vi "PID DAQ Multi-Channel UI Update.vi"(7 "Sample Data":dbl[][](array[numeric]), 8 "error in":errorcluster, 10 "Sample Parameter":variant[](array[variant]), 11 "Sample Number":i32) -> (0 "error out":errorcluster)   [LabVIEW 2011]
uses:
  Controls/User Interface Action.ctl
  Functional Global Data/Run Data.ctl
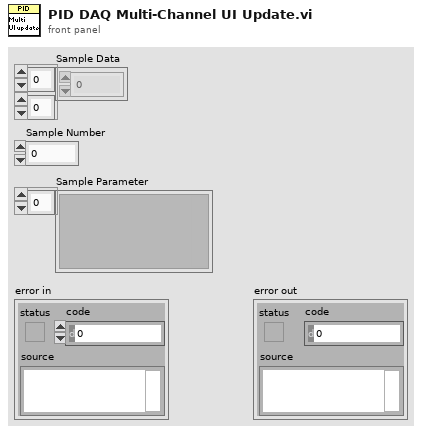
[diagram p1: front panel]
types:
  T1 = typedef "User Interface Action.ctl" = enum16{"Initialize", "Data Acquisition Disable", "Data View Disable", "Sample Set", "Sample Set 2D Data", "Sample Set x0 & dx", "Sample Add", "Sample Set Cursor", "Sample Set Offset & Multiplier", "Sample Set Axis Labels", "Sample Parameters Disabled", "Sample Parameters Update", "Run Update", "Run Set Offset & Multiplier", "Run Set Axis Labels", "Run Set Cursor", "Run Set Disabled", "Run Parameters Update", "Run Parameters Disabled", "Run Number Set", "Run Number Set Range", "Run Number Set Disabled", "Sample Number Set", "Sample Number Set Range", "Notes Set Value", "Update Plot", "Set Plot Parameters", "Update Concentration Plot", "Time Set", "Clear DAQ Display", "Clear Analysis Display", "Status Bar Set", "Progress Bar Set", "Display Mode Set", "Experiment Type Set", "Analysis Plot Average Set", "Stop"}
  T2 = typedef "Run Data.ctl" = enum16{"Initialize", "Add Sample Channel", "Set Run", "Get Number of Runs", "Set Run Params", "Get Spectrum", "Get Run Params", "Get Sample Params", "Get History", "Get Averaged History", "Get Run Param Names", "Set Run Param Names", "Get Sample Param Names", "Set Sample Param Names", "Get MFC Flow Rate Challenge Profile", "Get History Average"}
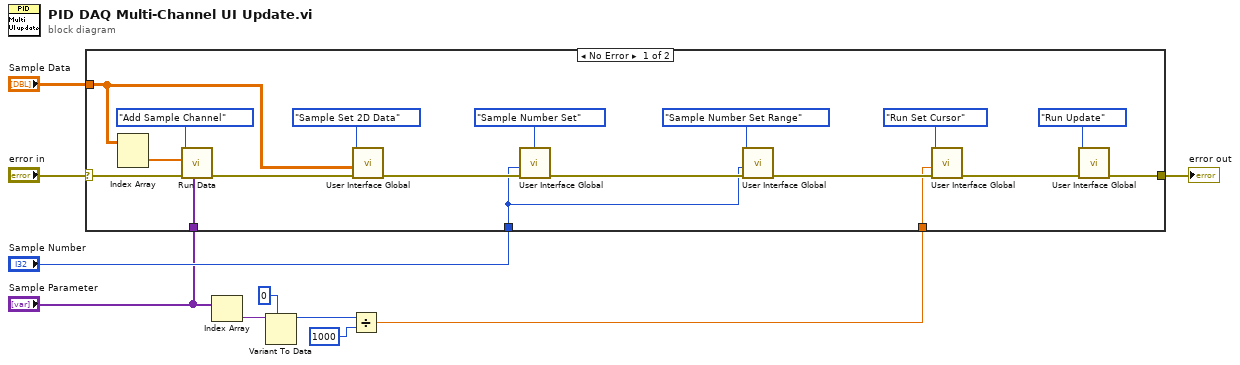
[diagram p0: block diagram]
diagram:
  n1 = Index Array(array="Sample Parameter") -> (element=w5:variant)  [unwired: 1 in]
  n2 = Variant To Data(type=0, Variant=w5) -> (data=w3:i32)  [unwired: 1 in, 1 out]
  n3 = Divide(x=w3, y=1000) -> (x/y=w1:dbl)
  n4 = case shown="No Error" "error in" {
    selector: "error in" -> [w19 w29]
    tunnel: [w13 w29] -> w10
    tunnel: "Sample Number" -> [w18 _]
    tunnel: "Sample Data" -> [w12 _]
    tunnel: "Sample Parameter" -> [w20 _]
    tunnel: w1 -> [w14 _]
    frame No Error {
      n5 = Index Array(array=w12) -> (element=w11:dbl[])  [unwired: 2 in]
      n6 = call "Run Data.vi"("Params 1D IN"=w20, "error in"=w19, "Data 1D IN"=w11, "action"=Run_Data."Add Sample Channel" ("Action")) -> ("error out"=w21:errorcluster)  [unwired: 4 in, 3 out]
      n7 = call "User Interface Global.vi"("error in"=w21, "data1"=w12, "action"=User_Interface_Action."Sample Set 2D Data" ("Action")) -> ("error out"=w27:errorcluster)  [unwired: 8 in]
      n8 = call "User Interface Global.vi"("error in"=w27, "data1"=w18, "action"=User_Interface_Action."Sample Number Set" ("Action")) -> ("error out"=w26:errorcluster)  [unwired: 8 in]
      n9 = call "User Interface Global.vi"("error in"=w26, "data1"=w18, "action"=User_Interface_Action."Sample Number Set Range" ("Action")) -> ("error out"=w16:errorcluster)  [unwired: 8 in]
      n10 = call "User Interface Global.vi"("error in"=w16, "data1"=w14, "action"=User_Interface_Action."Run Set Cursor" ("Action")) -> ("error out"=w15:errorcluster)  [unwired: 8 in]
      n11 = call "User Interface Global.vi"("error in"=w15, "action"=User_Interface_Action."Run Update" ("Action")) -> ("error out"=w13:errorcluster)  [unwired: 9 in]
    }
    frame Error {
    }
  }
  "error out" <- w10
